vi "array to test ver.1.0.vi"(1 "Values":bool[](array[boolean])=[FALSE, FALSE, FALSE, FALSE, FALSE, FALSE, FALSE, FALSE, FALSE, FALSE, FALSE, FALSE, FALSE, FALSE, FALSE, FALSE, FALSE, FALSE, FALSE, FALSE, FALSE, TRUE, FALSE, TRUE, FALSE, FALSE, FALSE, FALSE, FALSE, FALSE, FALSE, TRUE, FALSE, FALSE, FALSE]) -> (0 "output":string="~10000*100mV")   [LabVIEW 2021]
panel:
  out "number":u32=514
  out "val":i16=10000
  out "unit":bool[](array[boolean])=[FALSE, TRUE, FALSE, FALSE, FALSE, FALSE, FALSE, FALSE, FALSE, TRUE, FALSE, FALSE, FALSE]
  out "val":bool[](array[boolean])=[FALSE, FALSE, FALSE, FALSE, FALSE, FALSE, FALSE, FALSE, FALSE, FALSE, FALSE, FALSE, FALSE, FALSE, FALSE, FALSE, FALSE, FALSE, FALSE, TRUE]
  out "Array size":i32=35
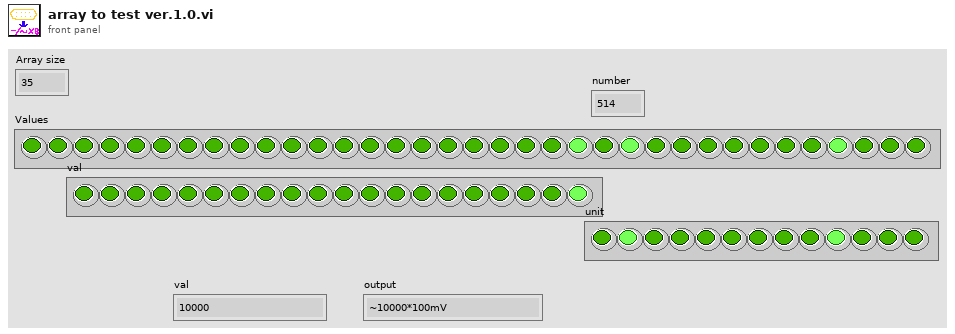
[diagram p1: front panel]
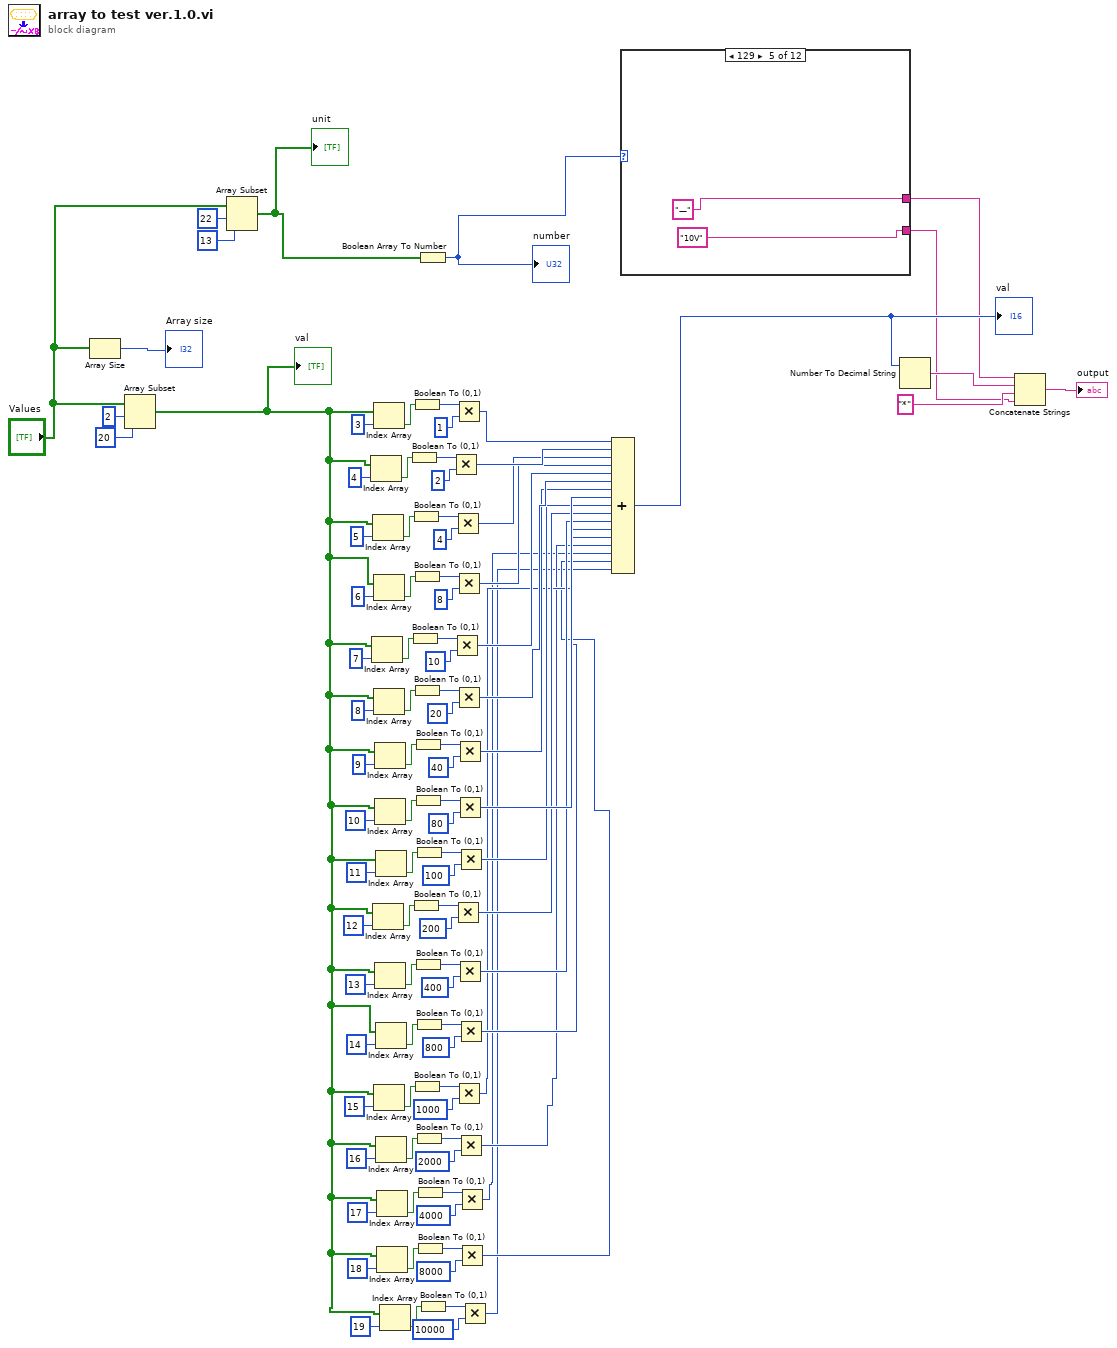
[diagram p0: block diagram]
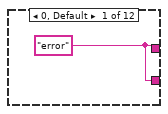
[diagram p2: hidden frame]
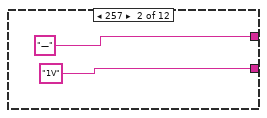
[diagram p3: hidden frame]
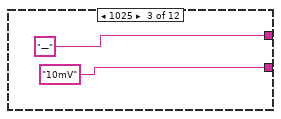
[diagram p4: hidden frame]
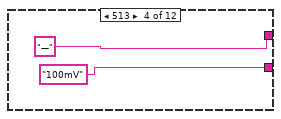
[diagram p5: hidden frame]
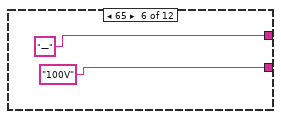
[diagram p6: hidden frame]
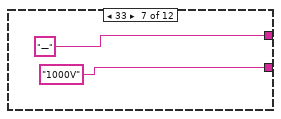
[diagram p7: hidden frame]
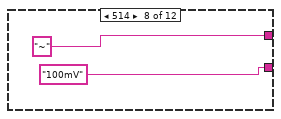
[diagram p8: hidden frame]
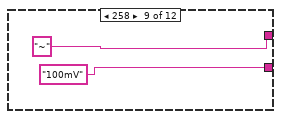
[diagram p9: hidden frame]
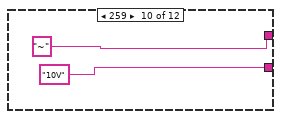
[diagram p10: hidden frame]
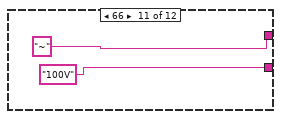
[diagram p11: hidden frame]
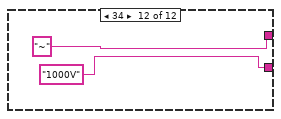
[diagram p12: hidden frame]
diagram:
  n1 = Array Size(array="Values") -> (size(s)=→"Array size":i32)
  n2 = Array Subset(array="Values", index=2 ("索引"), length=20 ("长度")) -> (w26:bool[])
  "val" <- w26
  n3 = Array Subset(array="Values", index=22 ("索引"), length=13 ("长度")) -> (w8:bool[])
  "unit" <- w8
  n4 = Index Array(array=w26, index=4 ("索引")) -> (element=w89:bool)
  n5 = Index Array(array=w26, index=7 ("索引")) -> (element=w77:bool)
  n6 = Index Array(array=w26, index=5 ("索引")) -> (element=w85:bool)
  n7 = Index Array(array=w26, index=12 ("索引")) -> (element=w57:bool)
  n8 = Index Array(array=w26, index=3 ("索引")) -> (element=w93:bool)
  n9 = Index Array(array=w26, index=6 ("索引")) -> (element=w81:bool)
  n10 = Index Array(array=w26, index=8 ("索引")) -> (element=w73:bool)
  n11 = Index Array(array=w26, index=15 ("索引")) -> (element=w45:bool)
  n12 = Index Array(array=w26, index=9 ("索引")) -> (element=w69:bool)
  n13 = Index Array(array=w26, index=10 ("索引")) -> (element=w65:bool)
  n14 = Index Array(array=w26, index=13 ("索引")) -> (element=w53:bool)
  n15 = Index Array(array=w26, index=11 ("索引")) -> (element=w61:bool)
  n16 = Index Array(array=w26, index=14 ("索引")) -> (element=w49:bool)
  n17 = Index Array(array=w26, index=16 ("索引")) -> (element=w41:bool)
  n18 = Index Array(array=w26, index=17 ("索引")) -> (element=w37:bool)
  n19 = Index Array(array=w26, index=18 ("索引")) -> (element=w33:bool)
  n20 = Index Array(array=w26, index=19 ("索引")) -> (element=w29:bool)
  n21 = Boolean To (0,1)(Boolean=w89) -> (0, 1=w88:i16)
  n22 = Boolean To (0,1)(Boolean=w77) -> (0, 1=w76:i16)
  n23 = Boolean To (0,1)(Boolean=w85) -> (0, 1=w84:i16)
  n24 = Boolean To (0,1)(Boolean=w57) -> (0, 1=w56:i16)
  n25 = Boolean To (0,1)(Boolean=w93) -> (0, 1=w92:i16)
  n26 = Boolean To (0,1)(Boolean=w81) -> (0, 1=w80:i16)
  n27 = Boolean To (0,1)(Boolean=w73) -> (0, 1=w72:i16)
  n28 = Boolean To (0,1)(Boolean=w45) -> (0, 1=w44:i16)
  n29 = Boolean To (0,1)(Boolean=w69) -> (0, 1=w68:i16)
  n30 = Boolean To (0,1)(Boolean=w65) -> (0, 1=w64:i16)
  n31 = Boolean To (0,1)(Boolean=w53) -> (0, 1=w52:i16)
  n32 = Boolean To (0,1)(Boolean=w61) -> (0, 1=w60:i16)
  n33 = Boolean To (0,1)(Boolean=w49) -> (0, 1=w48:i16)
  n34 = Boolean To (0,1)(Boolean=w41) -> (0, 1=w40:i16)
  n35 = Boolean To (0,1)(Boolean=w37) -> (0, 1=w36:i16)
  n36 = Boolean To (0,1)(Boolean=w33) -> (0, 1=w32:i16)
  n37 = Boolean Array To Number(Boolean array=w8) -> (number=w7:u32)
  "number" <- w7
  n38 = Boolean To (0,1)(Boolean=w29) -> (0, 1=w28:i16)
  n39 = Multiply(x=w88, y=i16 2) -> (x*y=w24:i16)
  n40 = Multiply(x=w76, y=i16 10) -> (x*y=w21:i16)
  n41 = Multiply(x=w84, y=i16 4) -> (x*y=w23:i16)
  n42 = Multiply(x=w56, y=i16 200) -> (x*y=w16:i16)
  n43 = Multiply(x=w92, y=i16 1) -> (x*y=w25:i16)
  n44 = Multiply(x=w80, y=i16 8) -> (x*y=w22:i16)
  n45 = Multiply(x=w72, y=i16 20) -> (x*y=w20:i16)
  n46 = Multiply(x=w44, y=i16 1000) -> (x*y=w13:i16)
  n47 = Multiply(x=w68, y=i16 40) -> (x*y=w19:i16)
  n48 = Multiply(x=w64, y=i16 80) -> (x*y=w18:i16)
  n49 = Multiply(x=w52, y=i16 400) -> (x*y=w15:i16)
  n50 = Multiply(x=w60, y=i16 100) -> (x*y=w17:i16)
  n51 = Multiply(x=w48, y=i16 800) -> (x*y=w14:i16)
  n52 = Multiply(x=w40, y=i16 2000) -> (x*y=w12:i16)
  n53 = Multiply(x=w36, y=i16 4000) -> (x*y=w11:i16)
  n54 = Multiply(x=w32, y=i16 8000) -> (x*y=w10:i16)
  n55 = Multiply(x=w28, y=i16 10000) -> (x*y=w9:i16)
  n56 = Compound Arithmetic op=ADD(w25, w24, w23, w22, w21, w20, w19, w18, w17, w16, w15, w14, w13, w12, w11, w10, w9) -> (w6:i16)
  "val" <- w6
  n57 = case shown="129" w7 {
    tunnel: [w101 "—" "—" "—" "—" "—" "—" "~" "~" "~" "~" "~"] -> w5
    tunnel: [w101 "1V" "10mV" "100mV" "10V" "100V" "1000V" "100mV" "100mV" "10V" "100V" "1000V"] -> w2
    frame 0, Default {
      w101 = "error"
    }
    frame 257 {
    }
    frame 1025 {
    }
    frame 513 {
    }
    frame 129 {
    }
    frame 65 {
    }
    frame 33 {
    }
    frame 514 {
    }
    frame 258 {
    }
    frame 259 {
    }
    frame 66 {
    }
    frame 34 {
    }
  }
  n58 = Number To Decimal String(number=w6) -> (decimal integer string=w4:string)  [unwired: 1 in]
  n59 = Concatenate Strings(w5, w4, "*" ("字符串"), w2) -> (→"output":string)
